vi "attenuation_comparator.vi"() -> ()   [LabVIEW 2021]
uses:
  <vilib>/Utility/file.llb/Read Delimited Spreadsheet (DBL).vi
panel:
  in  "Enum":T1(ring)=enum."Aire"
  out "Fracción de atenuación  2":cluster{"all rows":dbl[], "all rows":dbl[]}[](graph)=[{"all rows"=[0.001, 0.0015, 0.002, 0.003, 0.004, 0.005, 0.006, 0.008, 0.01, 0.015, 0.02, 0.03, 0.04, 0.05, 0.06, 0.08, 0.1, 0.15, 0.2, 0.3, 0.4, 0.5, 0.6, 0.8, 1.0, 1.25, 1.5, 2.0, 3.0, 4.0, 5.0, 6.0, 8.0, 10.0, 15.0, 20.0], "all rows"=[0.0, 0.0, 8.128610635378201e-269, 1.6772370249095521e-84, 1.1197028613988305e-36, 3.219148124309381e-19, 1.9905998449415737e-11, 3.1359290095472915e-05, 0.00484891650510377, 0.18768317070714904, 0.44503604504282124, 0.6868770289110291, 0.7646783431859415, 0.7970004783531054, 0.81391446365985, 0.8321854220086748, 0.8430744578744253, 0.8602777300074131, 0.8719702261321094, 0.8881629949163498, 0.8993347101080899, 0.9076739960832506, 0.9143334034742631, 0.9243633950226916, 0.9317227379741021, 0.9387275415233357, 0.9440841262660942, 0.9517812975946508, 0.9610873300491638, 0.9665425079273203, 0.970144742058198, 0.9726801270731399, 0.9760026279509255, 0.9780543870626683, 0.9807771611611423, 0.9820333597229952]}, {"all rows"=[0.001, 0.00104695, 0.0010961, 0.0010961, 0.0015, 0.002, 0.003, 0.004, 0.005, 0.006, 0.008, 0.0089789, 0.0089789, 0.01, 0.015, 0.02, 0.03, 0.04, 0.05, 0.06, 0.08, 0.1, 0.15, 0.2, 0.3, 0.4, 0.5, 0.6, 0.8, 1.0, 1.25, 1.5, 2.0, 3.0, 4.0, 5.0, 6.0, 8.0, 10.0, 15.0, 20.0], "all rows"=[0.0, 0.0, 0.0, 0.0, 0.0, 0.0, 0.0, 2.0543024849559518e-176, 8.629909517747027e-97, 3.3255680002078145e-59, 2.6105410816854122e-27, 4.2695560824512626e-20, 1.4684069595274868e-141, 6.074138869757453e-110, 3.472217829612268e-38, 8.068274750743429e-18, 2.991857876948909e-06, 0.00347119070927667, 0.047661925851377004, 0.15637060751844503, 0.41117251830107593, 0.5862878959684609, 0.7724127975596329, 0.8339412522931252, 0.8777959460902024, 0.8961543421301746, 0.9071925337825703, 0.9150139206474455, 0.9259500013649637, 0.9335741863260163, 0.9405597257540489, 0.9455908166897274, 0.9522003258635763, 0.9589453885176715, 0.9620892434116443, 0.9636706462654194, 0.9644454712542331, 0.9648274981655526, 0.9645016421941608, 0.9628852280101078, 0.9610811944872335]}]
  out "Coeficientes atenuacion  2":cluster{"all rows":dbl[], "all rows":dbl[]}(graph)={"all rows"=[0.001, 0.00104695, 0.0010961, 0.0010961, 0.0015, 0.002, 0.003, 0.004, 0.005, 0.006, 0.008, 0.0089789, 0.0089789, 0.01, 0.015, 0.02, 0.03, 0.04, 0.05, 0.06, 0.08, 0.1, 0.15, 0.2, 0.3, 0.4, 0.5, 0.6, 0.8, 1.0, 1.25, 1.5, 2.0, 3.0, 4.0, 5.0, 6.0, 8.0, 10.0, 15.0, 20.0], "all rows"=[10570.0, 9307.0, 8242.0, 9347.0, 4418.0, 2154.0, 748.8, 347.3, 189.9, 115.6, 52.55, 38.29, 278.4, 215.9, 74.05, 33.79, 10.92, 4.862, 2.613, 1.593, 0.763, 0.4584, 0.2217, 0.1559, 0.1119, 0.09413, 0.08362, 0.07625, 0.06605, 0.05901, 0.05261, 0.04803, 0.04205, 0.03599, 0.03318, 0.03177, 0.03108, 0.03074, 0.03103, 0.03247, 0.03408]}
  in  "Espesor (mm)":dbl=1.3
  in  "Material prueba":path=path "C:/Users/pbellido/Desktop/TEMAS PR_ALARA/COEFICIENTS_DATA/COBRE.txt"
  out "Fracción de atenuación":cluster{"all rows":dbl[], "all rows":dbl[]}(graph)={"all rows"=[0.001, 0.0015, 0.002, 0.003, 0.004, 0.005, 0.006, 0.008, 0.01, 0.015, 0.02, 0.03, 0.04, 0.05, 0.06, 0.08, 0.1, 0.15, 0.2, 0.3, 0.4, 0.5, 0.6, 0.8, 1.0, 1.25, 1.5, 2.0, 3.0, 4.0, 5.0, 6.0, 8.0, 10.0, 15.0, 20.0], "all rows"=[0.0, 0.0, 8.128610635378201e-269, 1.6772370249095521e-84, 1.1197028613988305e-36, 3.219148124309381e-19, 1.9905998449415737e-11, 3.1359290095472915e-05, 0.00484891650510377, 0.18768317070714904, 0.44503604504282124, 0.6868770289110291, 0.7646783431859415, 0.7970004783531054, 0.81391446365985, 0.8321854220086748, 0.8430744578744253, 0.8602777300074131, 0.8719702261321094, 0.8881629949163498, 0.8993347101080899, 0.9076739960832506, 0.9143334034742631, 0.9243633950226916, 0.9317227379741021, 0.9387275415233357, 0.9440841262660942, 0.9517812975946508, 0.9610873300491638, 0.9665425079273203, 0.970144742058198, 0.9726801270731399, 0.9760026279509255, 0.9780543870626683, 0.9807771611611423, 0.9820333597229952]}
  in  "espesor agua (mm)":dbl=10.0
  out "Coeficientes atenuacion agua":cluster{"all rows":dbl[], "all rows":dbl[]}(graph)={"all rows"=[0.001, 0.0015, 0.002, 0.003, 0.004, 0.005, 0.006, 0.008, 0.01, 0.015, 0.02, 0.03, 0.04, 0.05, 0.06, 0.08, 0.1, 0.15, 0.2, 0.3, 0.4, 0.5, 0.6, 0.8, 1.0, 1.25, 1.5, 2.0, 3.0, 4.0, 5.0, 6.0, 8.0, 10.0, 15.0, 20.0], "all rows"=[4078.0, 1376.0, 617.3, 192.9, 82.78, 42.58, 24.64, 10.37, 5.329, 1.673, 0.8096, 0.3756, 0.2683, 0.2269, 0.2059, 0.1837, 0.1707, 0.1505, 0.137, 0.1186, 0.1061, 0.09687, 0.08956, 0.07865, 0.07072, 0.06323, 0.05754, 0.04942, 0.03969, 0.03403, 0.03031, 0.0277, 0.02429, 0.02219, 0.01941, 0.01813]}
  in  "error in (no error)":errorcluster
  in  "Ruta  para el agua":path=path "C:/Users/pbellido/Desktop/TEMAS PR_ALARA/COEFICIENTS_DATA/WATER.txt"
  # "Datos Agua"
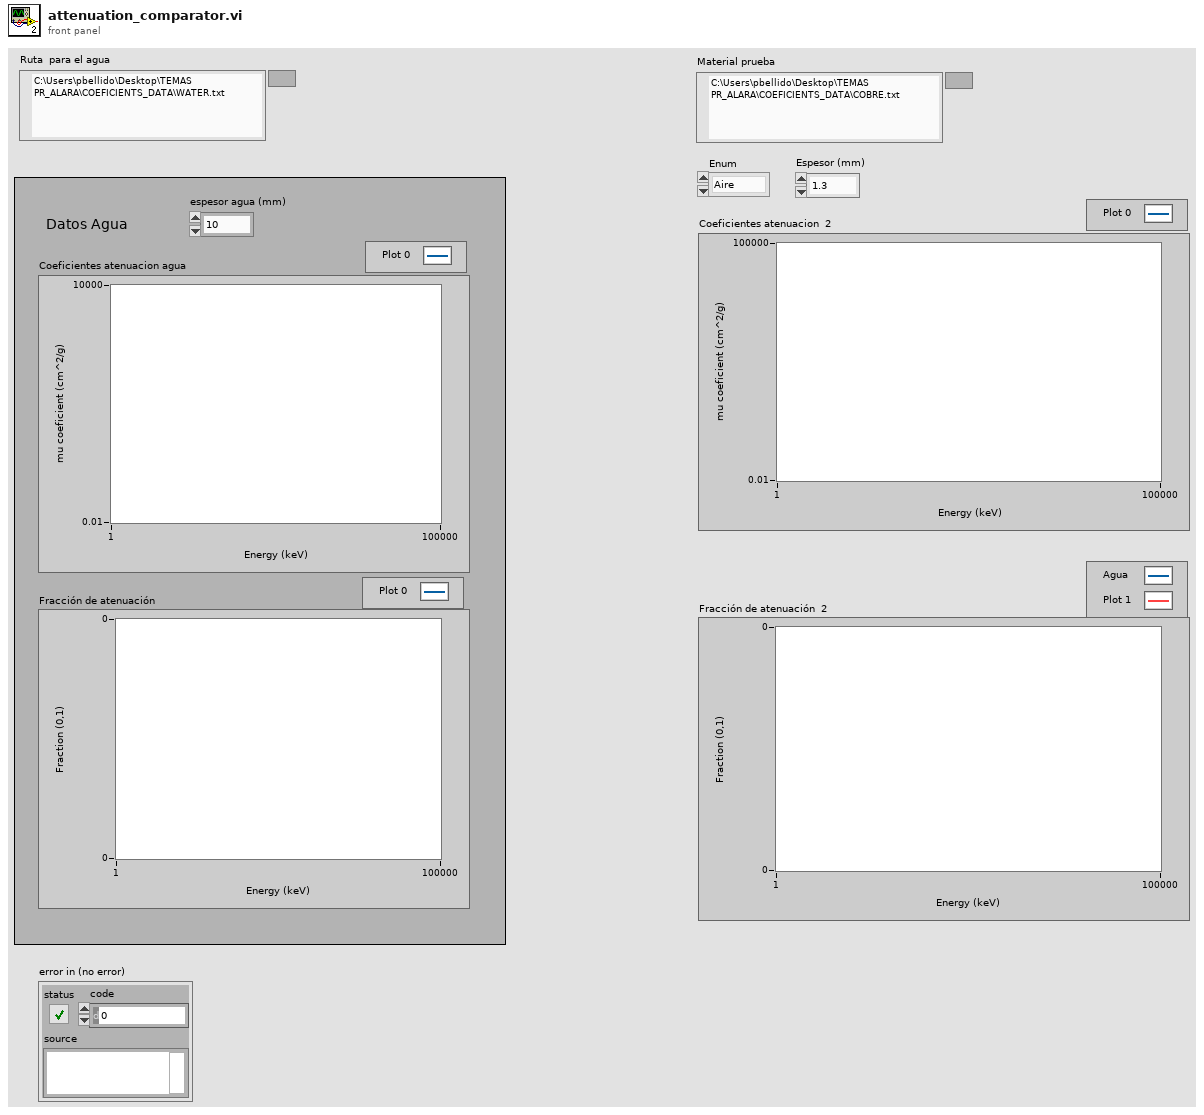
[diagram p1: front panel]
types:
  T1 = enum16{"Teflón", "Aluminio", "Plomo", "Aire", "Cobre"}
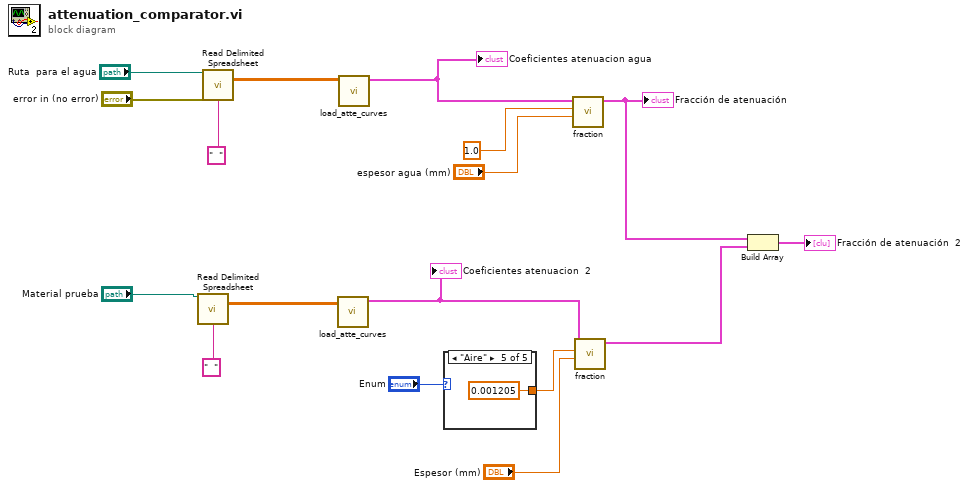
[diagram p0: block diagram]
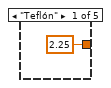
[diagram p2: hidden frame]
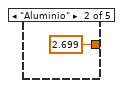
[diagram p3: hidden frame]
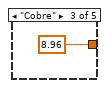
[diagram p4: hidden frame]
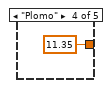
[diagram p5: hidden frame]
diagram:
  n1 = call-poly <vilib>:"Read Delimited Spreadsheet.vi"("file path (dialog if empty)"="Material prueba", "delimiter (\\t)"="  " ("delimiter (\\t)")) -> ("all rows"=w8:dbl[][])  [unwired: 8 in, 5 out]
  n2 = call-poly <vilib>:"Read Delimited Spreadsheet.vi"("file path (dialog if empty)"="Ruta  para el agua", "error in (no error)"="error in (no error)", "delimiter (\\t)"="  " ("delimiter (\\t)")) -> ("all rows"=w14:dbl[][])  [unwired: 7 in, 5 out]
  n3 = call "load_atte_curves.vi"("all rows"=w8) -> ("curva atenuation"=w5:cluster{"Energia":dbl[], "coeficiente":dbl[]})  [unwired: 10 in]
  "Coeficientes atenuacion  2" <- w5
  n4 = call "load_atte_curves.vi"("all rows"=w14) -> ("curva atenuation"=w11:cluster{"Energia":dbl[], "coeficiente":dbl[]})  [unwired: 10 in]
  "Coeficientes atenuacion agua" <- w11
  n5 = case shown="\"Aire\"" "Enum" {
    tunnel: [2.25 ("Densidad") 2.699 ("Densidad") 8.96 ("Densidad") 11.35 ("Densidad") 0.001205 ("Densidad")] -> w7
    frame "Teflón" {
    }
    frame "Aluminio" {
    }
    frame "Cobre" {
    }
    frame "Plomo" {
    }
    frame "Aire" {
    }
  }
  n6 = call "fraction.vi"("espesor"="espesor agua (mm)", "desnsidad"=1.0, "curva atenuation"=w11) -> ("Single Plot (X Array and Y Array) 2"=w4:cluster{"all rows":dbl[], "all rows":dbl[]})  [unwired: 8 in]
  "Fracción de atenuación" <- w4
  n7 = call "fraction.vi"("espesor"="Espesor (mm)", "desnsidad"=w7, "curva atenuation"=w5) -> ("Single Plot (X Array and Y Array) 2"=w3:cluster{"all rows":dbl[], "all rows":dbl[]})  [unwired: 8 in]
  n8 = Build Array(w4, w3) -> (→"Fracción de atenuación  2":cluster{"all rows":dbl[], "all rows":dbl[]}[])
